vi "plot.issues.vi"(5 "volume.volume type":T1 caption="Enum", 7 "volume_name":string, 8 "error in (no error)":errorcluster, 9 "cover_dates":timestamp[](array[timestamp]), 10 "issue_numbers":string[](array[string]), 11 "picture ref":refnum<vi>) -> (0 "error out":errorcluster, 3 "reference out":refnum<vi>)   [LabVIEW 2024]
uses:
  definitions/volume.type--enum.ctl
  volume.type.colors--cluster.ctl
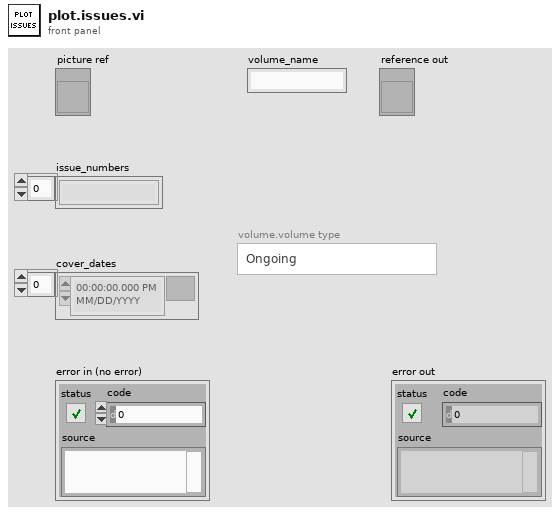
[diagram p1: front panel]
types:
  T1 = typedef "volume.type--enum.ctl" = enum16{"Ongoing", "Limited Series", "Annual", "One Shot", "Reprint/Document", "Star Comics", "Epic Comics"}
  T2 = typedef "volume.type.colors--cluster.ctl" = cluster{"ongoing":u32, "Limited Series":u32, "Annuals":u32, "One Shots":u32, "Reprints":u32, "Star":u32, "Epic":u32}
  T3 = cluster{"left":i16, "top":i16, "right":i16, "bottom":i16}
  T4 = cluster{"Time Stamp":timestamp, "String":string}[]
  T5 = typedef "LVBoundsTypeDef.ctl" = cluster{"Width":u32, "Height":u32}
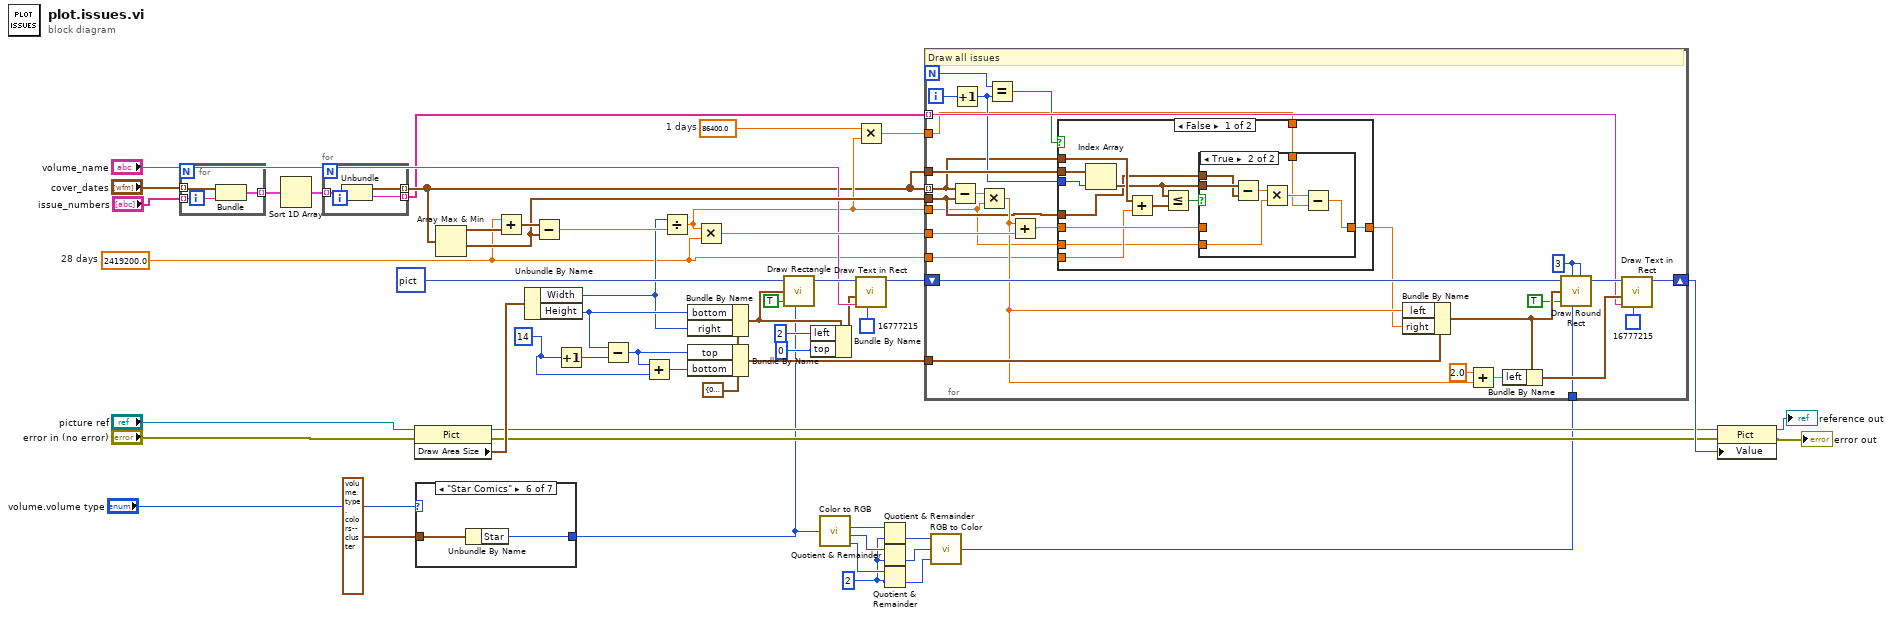
[diagram p0: block diagram]
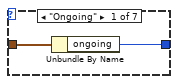
[diagram p2: hidden frame]
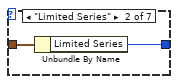
[diagram p3: hidden frame]
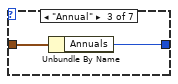
[diagram p4: hidden frame]
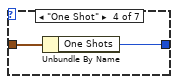
[diagram p5: hidden frame]
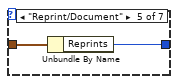
[diagram p6: hidden frame]
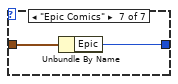
[diagram p7: hidden frame]
diagram:
  w10 = 86400.0  # 1 days
  w15 = u8 2 ("y")
  w37 = i16 14 ("y")
  w31 = T3 {"left"=0, "top"=0, "right"=0, "bottom"=0} ("rect")
  w7 = 2419200.0  # 28 days
  n1 = for {
    tunnel: "issue_numbers" -> [w55] mode=indexing
    tunnel: "cover_dates" -> [w54] mode=indexing
    tunnel: [w53] -> w6 mode=indexing
    n2 = Bundle("Time Stamp"=w54, "String"=w55) -> (w53:cluster{"Time Stamp":timestamp, "String":string})  [unwired: 1 in]
  }
  n3 = Sort 1D Array(array=w6) -> (sorted array=w5:T4)
  n4 = for {
    tunnel: w5 -> [w58] mode=indexing
    tunnel: [w57] -> w3 mode=indexing
    tunnel: [w56] -> w1 mode=indexing
    n5 = Unbundle(w58) -> ("Time Stamp"=w57:timestamp, "String"=w56:string)
  }
  n6 = property class="Pict"(reference="picture ref", error in="error in (no error)") -> (reference out=w43:refnum<vi>, error out=w42:errorcluster, "Draw Area Size"=w48:T5)
  n7 = case shown="\"Star Comics\"" "volume.volume type" {
    tunnel: T2 {"ongoing"=34559, "Limited Series"=35193, "Annuals"=16754450, "One Shots"=7566195, "Reprints"=16722176, "Star"=49407, "Epic"=7274696} ("Legend") -> [w60 w62 w64 w66 w68 w70 w72]
    tunnel: [w59 w61 w63 w65 w67 w69 w71] -> w19
    frame "Ongoing" {
      n8 = Unbundle By Name(w60) -> ("ongoing"=w59:u32)
    }
    frame "Limited Series" {
      n9 = Unbundle By Name(w62) -> ("Limited Series"=w61:u32)
    }
    frame "Annual" {
      n10 = Unbundle By Name(w64) -> ("Annuals"=w63:u32)
    }
    frame "One Shot" {
      n11 = Unbundle By Name(w66) -> ("One Shots"=w65:u32)
    }
    frame "Reprint/Document" {
      n12 = Unbundle By Name(w68) -> ("Reprints"=w67:u32)
    }
    frame "Star Comics" {
      n13 = Unbundle By Name(w70) -> ("Star"=w69:u32)
    }
    frame "Epic Comics" {
      n14 = Unbundle By Name(w72) -> ("Epic"=w71:u32)
    }
  }
  n15 = Array Max & Min(array=w3) -> (max value=w50:timestamp, min value=w46:timestamp)  [unwired: 2 out]
  n16 = Add(x=w7, y=w50) -> (x+y=w49:timestamp)
  n17 = Unbundle By Name(w48) -> ("Width"=w29:u32, "Height"=w30:u32)
  n18 = Subtract(x=w49, y=w46) -> (x-y=w47:dbl)
  n19 = Increment(x=w37) -> (x+1=w39:i16)
  n20 = Subtract(x=w30, y=w39) -> (x-y=w38:u32)
  n21 = Add(x=w38, y=w37) -> (x+y=w36:u32)
  n22 = Divide(x=w29, y=w47) -> (x/y=w9:dbl)
  n23 = Bundle By Name(cluster=w31, "bottom"=w30, "right"=w29) -> (w23:T3)
  n24 = Bundle By Name(cluster=w31, "top"=w38, "bottom"=w36) -> (w32:T3)
  n25 = Multiply(x=w9, y=w7) -> (x*y=w45:dbl)
  n26 = call <vilib>:"Draw Rectangle.vi"("picture"=picture data[5B], "rect"=w23, "fill?(F)"=TRUE, "color(black)"=w19) -> ("new picture"=w27:picture)  [unwired: 5 in]
  n27 = Bundle By Name(cluster=w23, "left"=i16 2, "top"=i16 0) -> (w24:T3)
  n28 = call <vilib>:"Color to RGB.vi"("Color"=w19) -> ("R"=w18:u8, "G"=w17:u8, "B"=w16:u8)  [unwired: 1 out]
  n29 = Multiply(x=w10, y=w9) -> (x*y=w8:dbl)
  n30 = call <vilib>:"Draw Text in Rect.vi"("text color(black)"=u32 16777215, "text"="volume_name", "rect"=w24, "picture"=w27) -> ("new picture"=w26:picture)  [unwired: 7 in]
  n31 = Quotient & Remainder(x=w18, y=w15) -> (floor(x/y)=w14:u8)  [unwired: 1 out]
  n32 = Quotient & Remainder(x=w17, y=w15) -> (floor(x/y)=w13:u8)  [unwired: 1 out]
  n33 = Quotient & Remainder(x=w16, y=w15) -> (floor(x/y)=w12:u8)  [unwired: 1 out]
  n34 = call <vilib>:"RGB to Color.vi"("B"=w12, "G"=w13, "R"=w14) -> ("Color"=w11:u32)
  n35 = for {
    N -> [w83]
    tunnel: w9 -> [w74]
    tunnel: w46 -> [w75]
    tunnel: w45 -> [w99]
    tunnel: w32 -> [w98]
    shift-right: [w89] -> w44
    shift-left: w26 -> [w97]
    tunnel: w1 -> [w86] mode=indexing
    tunnel: w3 -> [w76] mode=indexing
    tunnel: w11 -> [w85]
    tunnel: w3 -> [w79]
    tunnel: w8 -> [w73]
    tunnel: w7 -> [w77]
    i -> [w84]
    w96 = i16 3 ("oval width")
    # "Draw all issues"
    n36 = Subtract(x=w76, y=w75) -> (x-y=w100:dbl)
    n37 = Increment(x=w84) -> (x+1=w78:i32)
    n38 = Multiply(x=w100, y=w74) -> (x*y=w95:dbl)
    n39 = Equal?(x=w83, y=w78) -> (x = y?=w82:bool)
    n40 = Add(x=w95, y=w99) -> (x+y=w80:dbl)
    n41 = case shown="False" w82 {
      tunnel: [w109 w121] -> w81
      tunnel: w80 -> [w108 w121]
      tunnel: w79 -> [w112 _]
      tunnel: w78 -> [w111 _]
      tunnel: w77 -> [w107 _]
      tunnel: w76 -> [w105 _]
      tunnel: w75 -> [w103 _]
      tunnel: w74 -> [w102 _]
      tunnel: w73 -> [w101 _]
      frame False {
        n42 = Index Array(array=w112, index=w111) -> (element=w104:timestamp)
        n43 = Add(x=w105, y=w107) -> (x+y=w106:timestamp)
        n44 = Less Or Equal?(x=w104, y=w106) -> (x <= y?=w110:bool)
        n45 = case shown="True" w110 {
          tunnel: [w113 w114] -> w109
          tunnel: w108 -> [w113 _]
          tunnel: w104 -> [_ w120]
          tunnel: w103 -> [_ w119]
          tunnel: w102 -> [_ w117]
          tunnel: w101 -> [_ w115]
          frame False {
          }
          frame True {
            n46 = Subtract(x=w120, y=w119) -> (x-y=w118:dbl)
            n47 = Multiply(x=w118, y=w117) -> (x*y=w116:dbl)
            n48 = Subtract(x=w116, y=w115) -> (x-y=w114:dbl)
          }
        }
      }
      frame True {
      }
    }
    n49 = Bundle By Name(cluster=w98, "left"=w95, "right"=w81) -> (w92:T3)
    n50 = Add(x=2.0, y=w95) -> (x+y=w93:dbl)
    n51 = Bundle By Name(cluster=w92, "left"=w93) -> (w88:T3)
    n52 = call <vilib>:"Draw Round Rect.vi"("picture"=w97, "oval width"=w96, "rect"=w92, "fill?(F)"=TRUE, "color(black)"=w85, "oval height"=w96) -> ("new picture"=w90:picture)  [unwired: 3 in]
    n53 = call <vilib>:"Draw Text in Rect.vi"("text color(black)"=u32 16777215, "text"=w86, "rect"=w88, "picture"=w90) -> ("new picture"=w89:picture)  [unwired: 7 in]
  }
  n54 = property class="Pict"(reference=w43, error in=w42, "Value"=w44) -> (reference out=→"reference out":refnum<vi>, error out=→"error out":errorcluster)
